vi "AddUpdateEvent.vi"(8 "error in (no error)":errorcluster, 10 "UpdateEvent":refnum<user-event>, 11 "reference in":refnum<class "Switch_MotorP5.lvclass">) -> (0 "error out":errorcluster, 3 "reference in":refnum<class "Switch_MotorP5.lvclass">)   [LabVIEW 2022 SP3, in "Switch_MotorP5.lvlib" / "Switch_MotorP5.lvclass"]
uses:
  Switch_MotorP5.lvclass
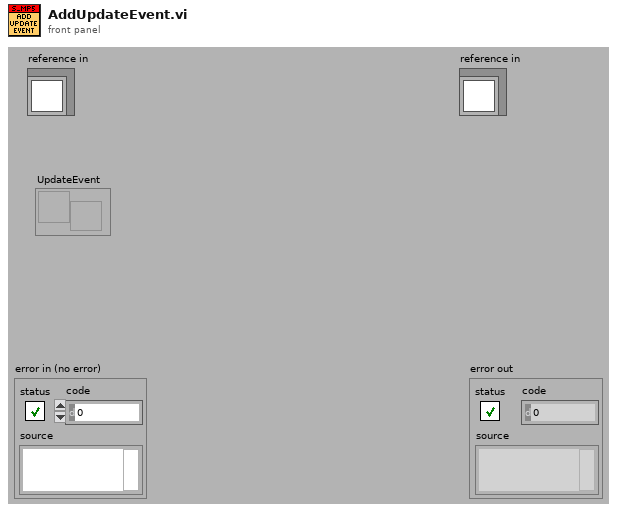
[diagram p1: front panel]
types:
  T1 = typedef "Switch_MotorP5.lvlib/Switch_MotorP5.lvclass/ObjectAttributes.ctl" = cluster{"Config":T2, "VISA":refnum<visa-resource-name>, "RPM":i32, "States":bool[], "UpdateEvent":refnum<user-event>, "Motor":enum32{"M1", "M2", "M3", "M4", "M5", "M6", "M7", "M8"}}
  T2 = typedef "Switch_MotorP5.lvlib/Switch_MotorP5.lvclass/Config.ctl" = cluster{"COM":refnum<visa-resource-name>, "SwitchMap":cluster{"Name":string, "Description":string, "Group":string, "IsGroup":bool, "Motor":enum32{"M1", "M2", "M3", "M4", "M5", "M6", "M7", "M8", "NA"}}[], "Sim":bool}
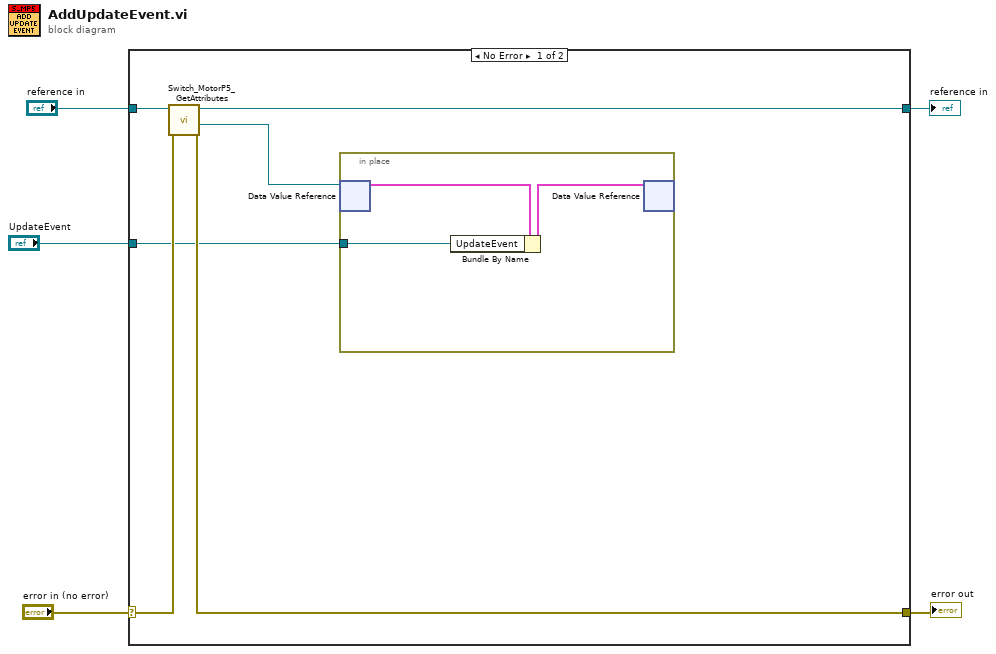
[diagram p0: block diagram]
diagram:
  n1 = case shown="No Error" "error in (no error)" {
    selector: "error in (no error)" -> [w11 w16]
    tunnel: [w10 w16] -> w4
    tunnel: [w8 w15] -> w2
    tunnel: "reference in" -> [w9 w15]
    tunnel: "UpdateEvent" -> [w6 _]
    frame No Error {
      n2 = call "Switch_MotorP5_GetAttributes.vi"("error in (no error)"=w11, "reference in"=w9) -> ("error out"=w10:errorcluster, "DataRef"=w7:refnum<data-value>, "reference out"=w8:refnum<class "Switch_MotorP5.lvclass">)  [unwired: 6 in, 1 out]
      n3 = in-place {
        in-place-border: w6 -> [w12]
        n4 = in-place-dvr #1(w7) -> (w14:T1)  [unwired: 1 out]
        n5 = Bundle By Name(cluster=w14, "UpdateEvent"=w12) -> (w13:T1)
        n6 = in-place-dvr #1(w13) -> ()  [unwired: 2 out]
      }
    }
    frame Error {
    }
  }
  "error out" <- w4
  "reference in" <- w2
